vi "Read Addr.vi"(8 "error in (no error)":errorcluster, 11 "Lesker Pressure in":refnum<class "Lesker Pressure.lvclass">) -> (0 "error out":errorcluster, 2 "Addr":string, 3 "Lesker Pressure out":refnum<class "Lesker Pressure.lvclass">)   [LabVIEW 2022 SP3, in "Lesker Pressure.lvclass"]
uses:
  Lesker Pressure.lvclass
  Lesker Pressure.lvclass/Lesker Pressure.ctl
  Pressure Monitor.lvclass
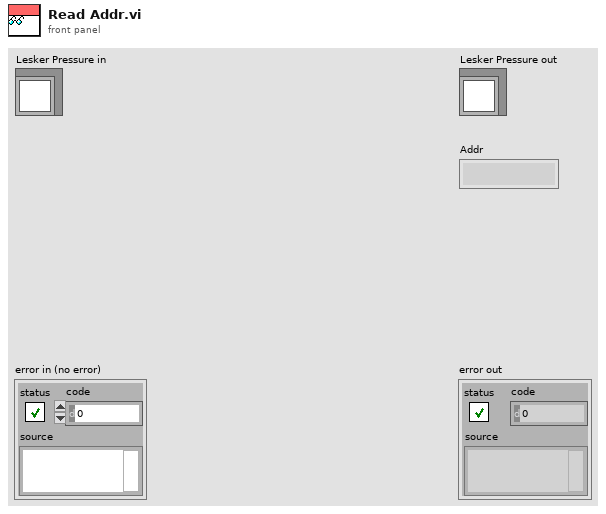
[diagram p1: front panel]
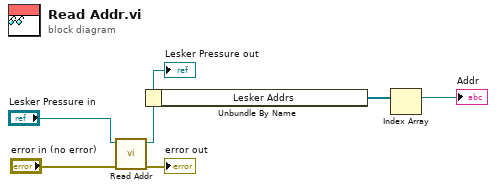
[diagram p0: block diagram]
diagram:
  n1 = call-parent "Read Addr.vi"("error in (no error)"="error in (no error)", "Pressure Monitor in"="Lesker Pressure in") -> ("error out"=→"error out":errorcluster, "Pressure Monitor out"=w3:refnum<class "Lesker Pressure.lvclass">)  [unwired: 7 in, 1 out]
  "Lesker Pressure out" <- w3
  n2 = Unbundle By Name(w3) -> ("Lesker Addrs"=w2:refnum<visa-resource-name>[])
  n3 = Index Array(array=w2) -> (element=→"Addr":refnum<visa-resource-name>)  [unwired: 1 in]
